vi "Add DI Coil.vi"(8 "error in (no error)":errorcluster, 9 "Mapping":T1={"DataType"=enum."U16", "Starting Address"=0, "Sub-Index (Bool)"=0, "VS Reference"=0}, 10 "Label":string="Discrete Input", 11 "Node Ref In":T3 format="%.0x") -> (0 "error out":errorcluster, 2 "Channel Ref Out":T3 format="%.0x", 3 "Node Ref out":T3 format="%.0x")   [LabVIEW 2015, in "Modbus Master System Explorer.lvlib"]
uses:
  Modbus Master System Explorer.lvlib
  <vilib>/NI Veristand/Custom Device API/Custom Device Item Ref.ctl
  Shared/Controls/Data Model/Mapping.ctl
  Shared/Controls/Data Model/DataType.ctl
  <vilib>/NI Veristand/Custom Device API/Custom Device Channel.ctl
  <vilib>/NI Veristand/Custom Device API/Custom Device Channel Type.ctl
  Modbus Type.ctl
  Radix.ctl
  Shared/Constants.vi
  <vilib>/NI VeriStand/Custom Device API/Custom Device API.lvlib
  Shared/Modbus Master Shared.lvlib
  <vilib>/NI VeriStand/Custom Device Tools/Custom Device Utility Library/Custom Device Utility Library.lvlib
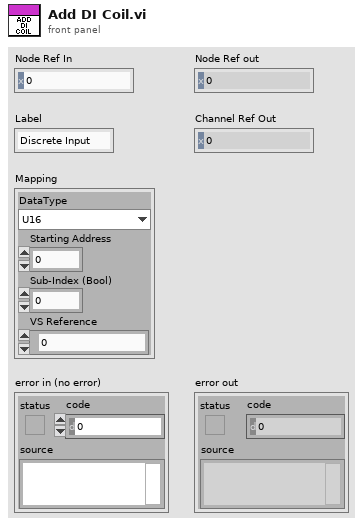
[diagram p1: front panel]
types:
  T1 = typedef "Modbus Master Shared.lvlib/Mapping.ctl" = cluster{"DataType":T2, "Starting Address":u16, "Sub-Index (Bool)":u16, "VS Reference":T3}
  T2 = typedef "Modbus Master Shared.lvlib/DataType.ctl" = enum16{"Double", "Single", "I64", "I32", "I16", "I8", "U64", "U32", "U16", "U8", "Boolean"}
  T3 = typedef "Custom Device API.lvlib/Custom Device Item Ref.ctl" = u64
  T4 = typedef "Modbus Master System Explorer.lvlib/Radix.ctl" = enum32{"Decimal", "Hexidecimal"}
  T5 = typedef "Custom Device API.lvlib/Custom Device Channel Type.ctl" = enum16{"Input", "Output"}
  T6 = typedef "Modbus Master Shared.lvlib/Modbus Type.ctl" = enum16{"Coil", "Discrete Input", "Holding Register", "Input Register"}
  T7 = typedef "Custom Device API.lvlib/Custom Device Channel.ctl" = cluster{"Type":T5, "Units":string, "Default Value":dbl, "Faultable":bool, "Scalable":bool}
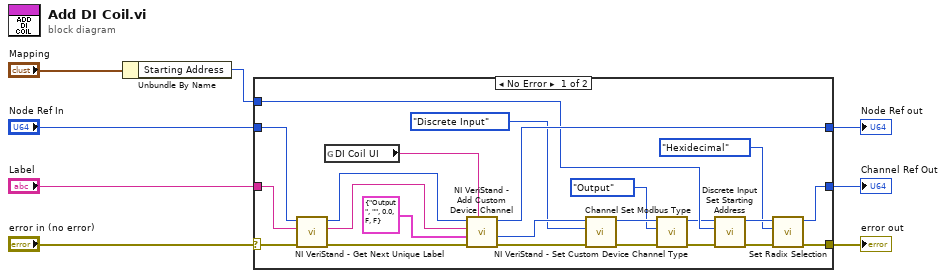
[diagram p0: block diagram]
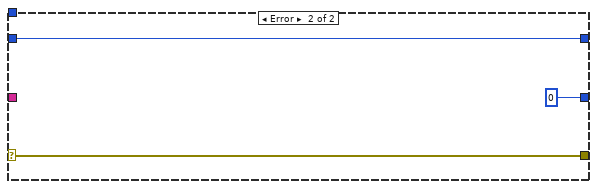
[diagram p2: hidden frame]
diagram:
  n1 = Unbundle By Name("Mapping") -> ("Starting Address"=w1:u16)
  n2 = case shown="No Error" "error in (no error)" {
    selector: "error in (no error)" -> [w25 w33]
    tunnel: "Node Ref In" -> [w27 w34]
    tunnel: [w10 w33] -> w6
    tunnel: [w24 w34] -> w5
    tunnel: [w12 T3 0 ("Channel Ref")] -> w4
    tunnel: "Label" -> [w23 _]
    tunnel: w1 -> [w22 _]
    frame No Error {
      n3 = call <vilib>:"NI VeriStand - Get Next Unique Label.vi"("error in (no error)"=w25, "Label"=w23, "Parent Ref in"=w27) -> ("error out"=w29:errorcluster, "Label out"=w30:string, "Parent Ref dup"=w28:T3)  [unwired: 5 in, 1 out]
      n4 = global read "Constants.vi" "DI Coil UI"() -> (w26:string)
      n5 = call <vilib>:"NI VeriStand - Add Custom Device Channel.vi"("GUID (Default Channel)"=w26, "error in (no error)"=w29, "Channel"=T7 {"Type"=enum."Output", "Units"="", "Default Value"=0.0, "Faultable"=FALSE, "Scalable"=FALSE}, "Channel Name"=w30, "Parent Ref in"=w28) -> ("error out"=w21:errorcluster, "Channel Ref"=w20:T3, "Parent Ref out"=w24:T3)  [unwired: 3 in, 1 out]
      n6 = call "Channel Set Modbus Type.vi"("error in (no error)"=w21, "Type"=Modbus_Type."Discrete Input", "Channel Ref"=w20) -> ("error out"=w15:errorcluster, "Item Ref out"=w18:T3)  [unwired: 7 in]
      n7 = call <vilib>:"NI VeriStand - Set Custom Device Channel Type.vi"("error in (no error)"=w15, "Type"=Custom_Device_Channel_Type."Output", "Channel Ref in"=w18) -> ("error out"=w14:errorcluster, "Channel Ref out"=w17:T3)  [unwired: 7 in]
      n8 = call "Discrete Input Set Starting Address.vi"("error in (no error)"=w14, "Value"=w22, "Item Ref in"=w17) -> ("error out"=w11:errorcluster, "Item Ref out"=w13:T3)  [unwired: 7 in]
      n9 = call "Set Radix Selection.vi"("error in (no error)"=w11, "Radix"=Radix."Hexidecimal", "Item Ref in"=w13) -> ("error out"=w10:errorcluster, "Item Ref out"=w12:T3)  [unwired: 7 in]
    }
    frame Error {
    }
  }
  "error out" <- w6
  "Node Ref out" <- w5
  "Channel Ref Out" <- w4
